vi "VescSetRpm.vi"(10 "error in (no error)":errorcluster, 11 "Speed (rpm)":i32) -> (3 "error out":errorcluster)   [LabVIEW 2019]
uses:
  <vilib>/myRIO/Instrument Drivers/Onboard IO/UART/typedef/VISA Configuration.ctl
  <vilib>/Instr/_visa.llb/VISA Configure Serial Port (Instr).vi
  <vilib>/myRIO/Express VI/Onboard IO/UART/UART Express VI.xnode
  <vilib>/myRIO/Instrument Drivers/Onboard IO/UART/UART.lvlib
  libvescEncoder.dll
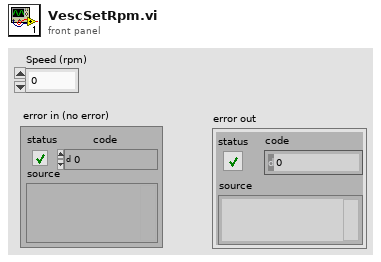
[diagram p1: front panel]
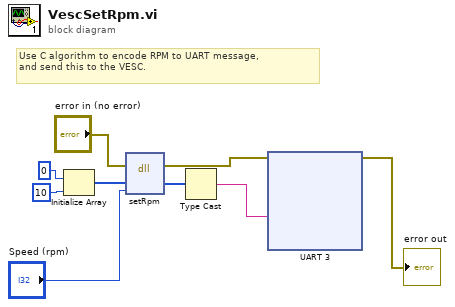
[diagram p0: block diagram]
diagram:
  # "Use C algorithm to encode RPM to UART message,\nand send this to the VESC."
  n1 = Initialize Array(0, 10) -> (w7:i32[])
  n2 = dll-call lib="libvescEncoder.*" fn="setRpm"(error in="error in (no error)", "array"=w7, "rpm"="Speed (rpm)") -> (error out=w3:errorcluster, "array"=w6:u8[])  [unwired: 4 in, 1 out]
  n3 = Type Cast(x=w6) -> (*(type *) &x=w2:string)  [unwired: 1 in]
  n4 = xnode "UART 3"("Characters to Write"=w2, "error in (no error)"=w3) -> ("error out"=→"error out":errorcluster)  [unwired: 1 out]
